vi "Pressure Tapped wing.vi"() -> ()   [LabVIEW 2022 SP3]
uses:
  Anemometry/Anemometry Sub Vis/Controls/User_Specific_mode.ctl
  Anemometry/Anemometry Sub Vis/Gen Trav/Trav_mode.ctl
  Anemometry/Anemometry Sub Vis/Controls/Tunnel_Coordinates.ctl
  Anemometry/Anemometry Sub Vis/Controls/Save_Data.ctl
  Anemometry/Anemometry Sub Vis/Gen Trav/Spacing.ctl
  Anemometry/Anemometry Sub Vis/Controls/Multi_run_mode.ctl
  Anemometry/Anemometry Sub Vis/Gen Trav/Traverse_cluster.ctl
  ADAM Client/Sub VIs/ADAM Controls/Tunnel_speed_mode.ctl
panel:
  in  "Tunnel Speed":dbl
  in  "End Position (mm)":sgl
  in  "Angle of Attack":sgl format="%#.1f"
  in  "Zero Pressure Transducers":bool
  in  "Take Traverse Profile":bool
  out "Velocity Profile":cluster{dbl[], dbl[]}(graph)
  in  "stop":bool
  out "Currently on Point":i32
  in  "Measure Pressures\n(without Saving)":bool
  in  "Number of Points":i32
  in  "Start Position (mm)":sgl
  out "Z":dbl format="%#.0f"
  out "U Trav":dbl format="%.2f"
  out "Uref":dbl format="%.2f"
  out "Pressure Distribution over wing":cluster{dbl[], dbl[]}[](graph)
  in  "Averaging time (Sec)":dbl=5.0
  in  "Filename":path=path "\\\\surrey.ac.uk\\personal/HS103/m13602/Documents/Wing_Results/test1.xls"
  in  "Take Pressure Measurement":bool
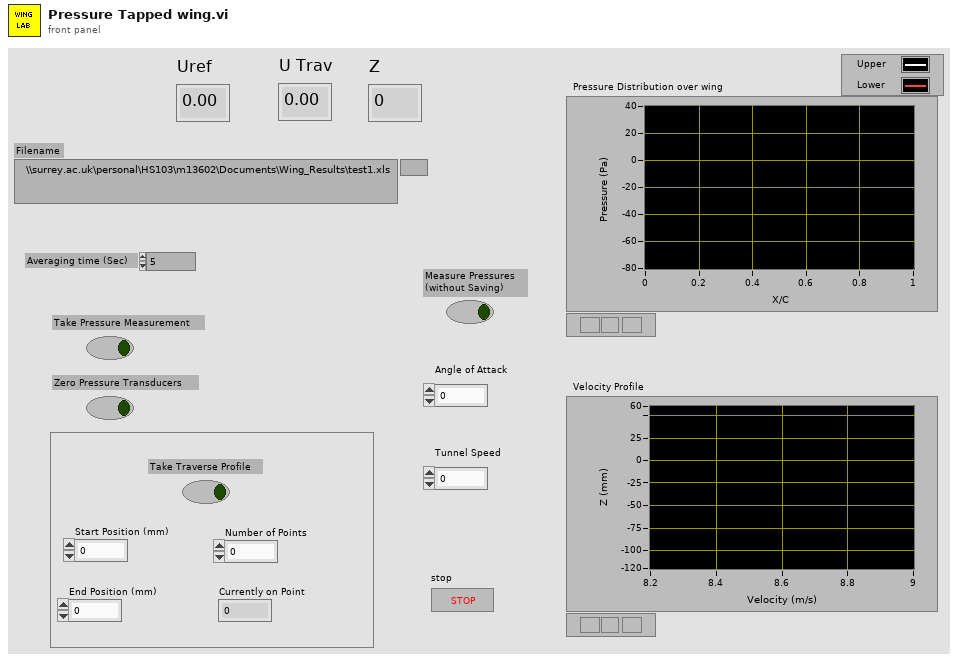
[diagram p1: front panel]
types:
  T1 = typedef "Tunnel_speed_mode.ctl" = enum16{"Set Speed", "Set Speed then wait", "Is tunnel speed allowable?"}
  T2 = typedef "Trav_mode.ctl" = enum16{"Move traverse", "Read traverse position", "Teach Position"}
  T3 = typedef "Tunnel_Coordinates.ctl" = enum16{"Work in Tunnel Coordinates", "Work in Model Coordinates"}
  T4 = typedef "User_Specific_mode.ctl" = enum16{"Check VI only", "Run VI"}
  T5 = typedef "Save_Data.ctl" = enum16{"Save No Data", "Save Data"}
  T6 = typedef "Traverse_cluster.ctl" = cluster{"Start X":sgl, "Start Y":sgl, "Start Z":sgl, "End X":sgl, "End Y":sgl, "End Z":sgl, "nPoints":i32, "Spacing":T7, "Filename":path, "Tunnel Speed":dbl, "Averaging time (mins)":dbl, "Extra Commands":string, "Carrier_1 Q (l/min)":dbl, "Carrier_2 Q (l/min)":dbl, "Trace Gas Concentration (%)":dbl, "Specific Arguments":string, "Comments":string, "Row No":i32, "Row Type Selector":T8, "EstCompl":string, "Row Duration (mins)":dbl, "nValidPoints":i32, "Meas Setup File":string}
  T7 = typedef "Spacing.ctl" = enum16{"Linear", "Log", "Gauss", "Specified", "N/A"}
  T8 = typedef "Multi_run_mode.ctl" = enum16{"Move Traverse Only", "Set Tunnel Speed Only", "Set Source Only", "Set Measurement Conditions", "Single Measurement", "Vertical Profile", "Lateral Profile", "Longitudinal Profile", "Multi-Axis Profile", "Explore Volume", "Auto Calibrate", "Meas Fast FID Bkgnd", "Check Beam Power", "Scanning Valve Measurement", "Run VI Named:", "Set ADAM Ch", "Wait (minutes)", "Send Message", "Synchronize With:", "Fall Back to this Row", "Turn Off Row Repeating", "Traverse 3D Volume", "Blank Row", "Jump to Fall Back Row"}
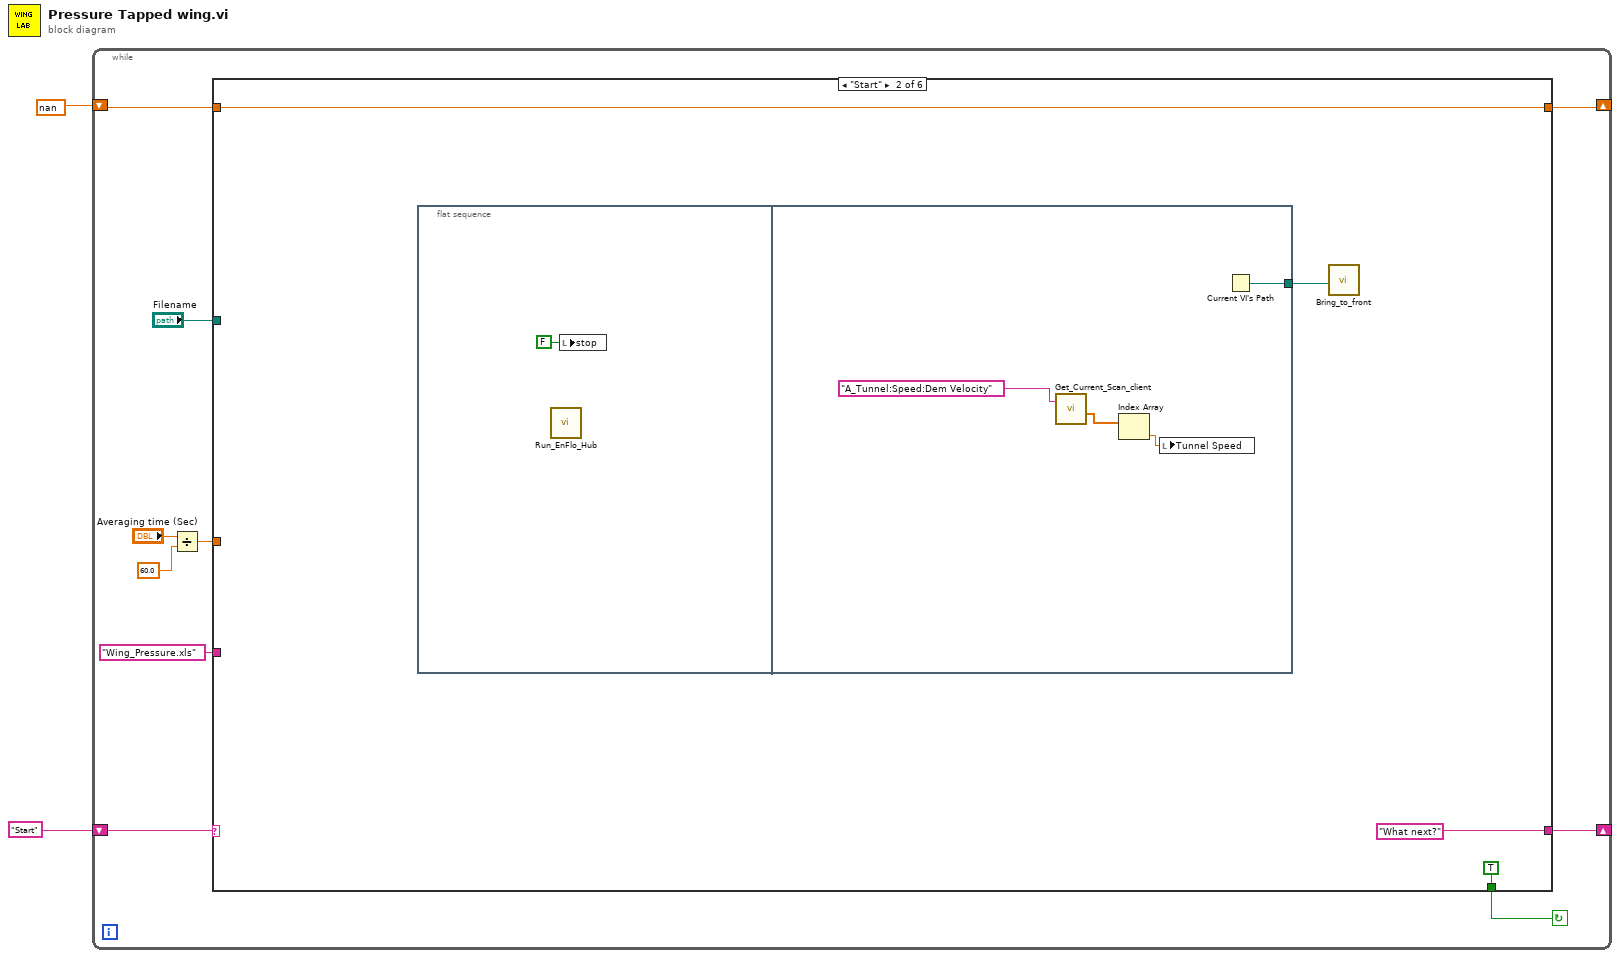
[diagram p0: block diagram]
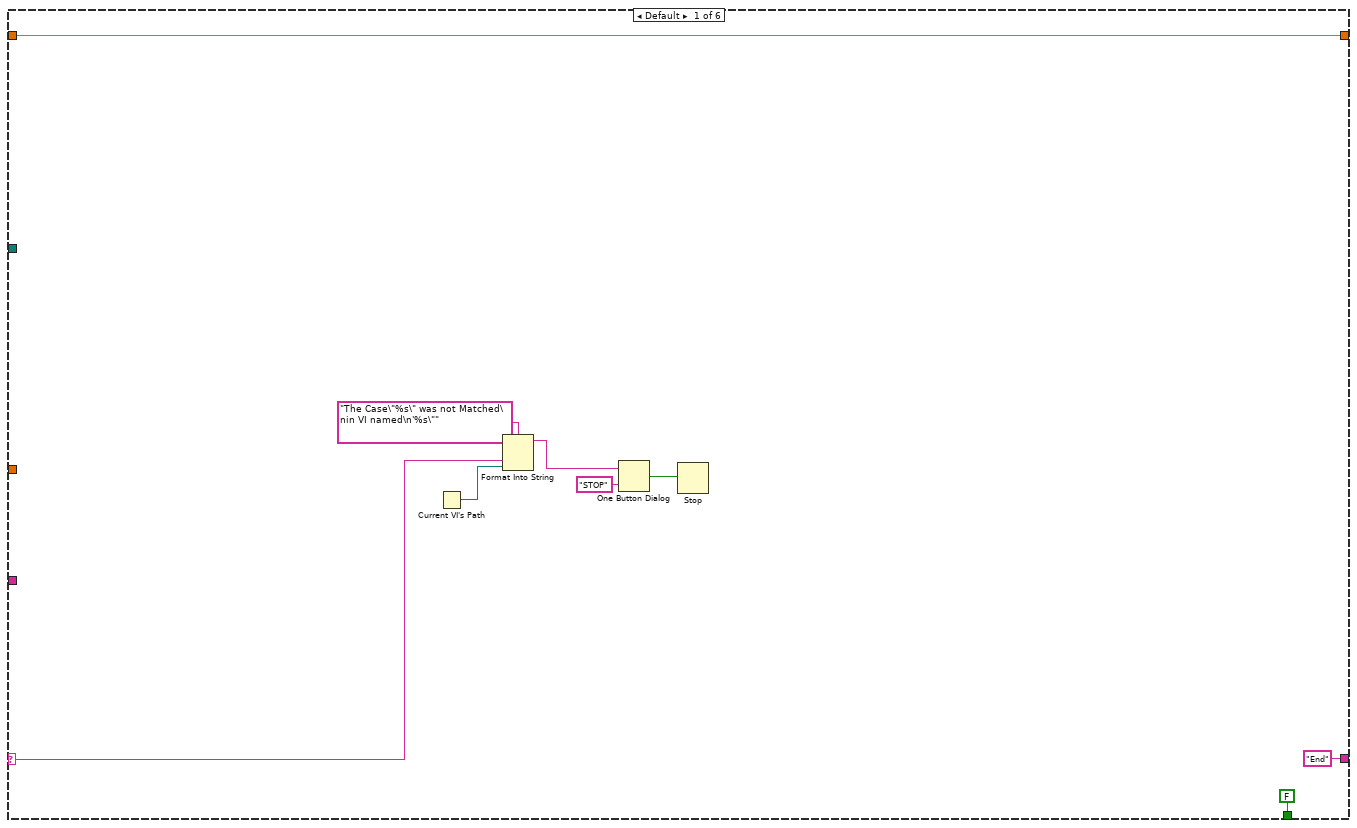
[diagram p2: hidden frame]
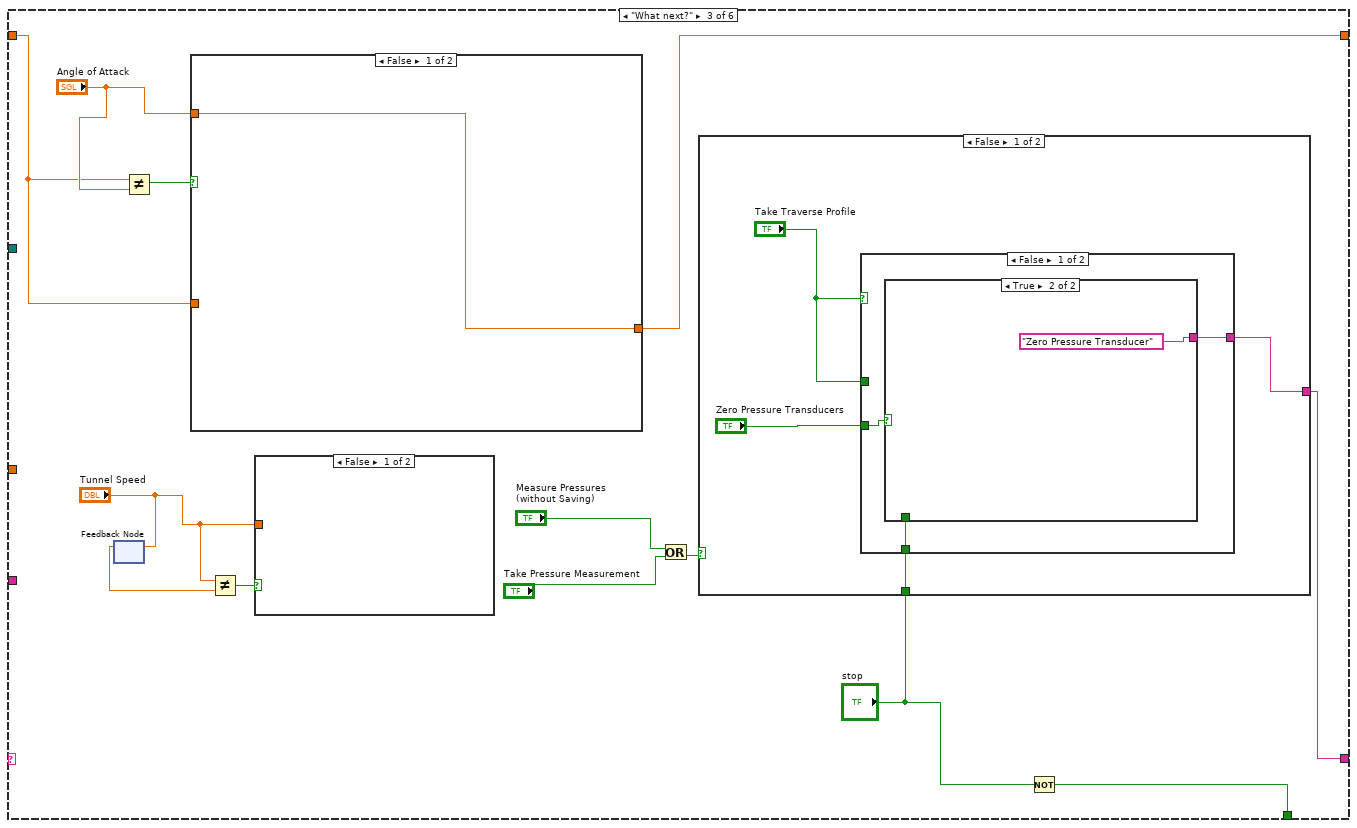
[diagram p3: hidden frame]
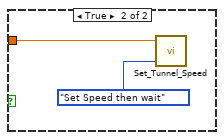
[diagram p4: hidden frame]
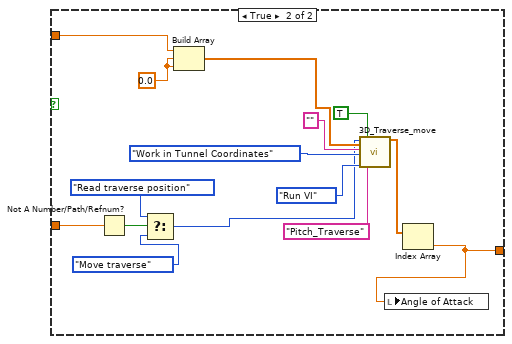
[diagram p5: hidden frame]
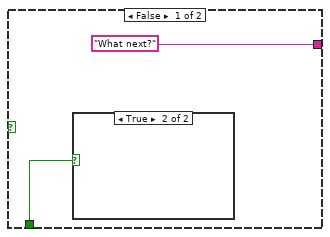
[diagram p6: hidden frame]
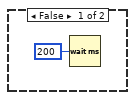
[diagram p7: hidden frame]
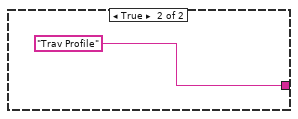
[diagram p8: hidden frame]
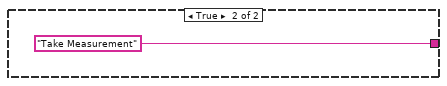
[diagram p9: hidden frame]
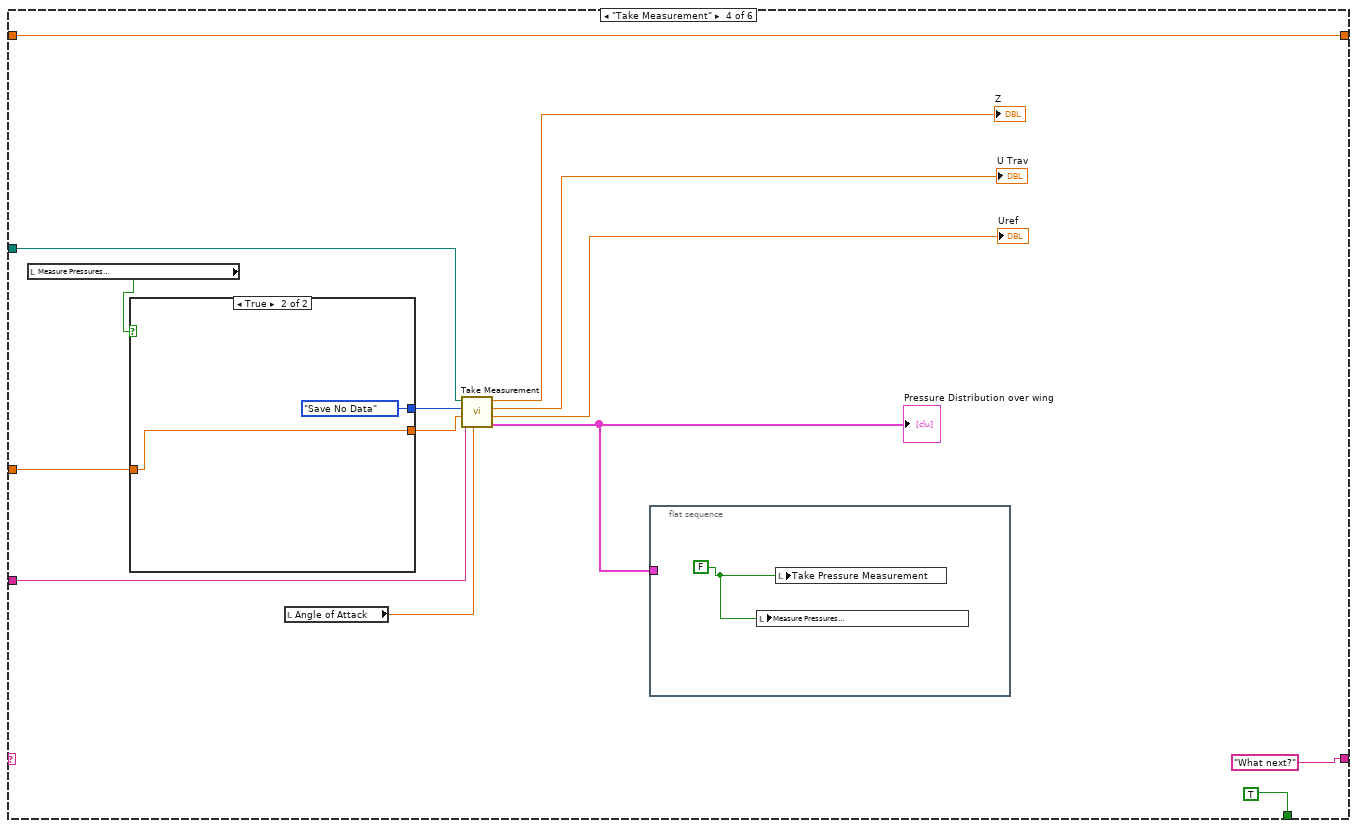
[diagram p10: hidden frame]
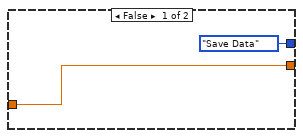
[diagram p11: hidden frame]
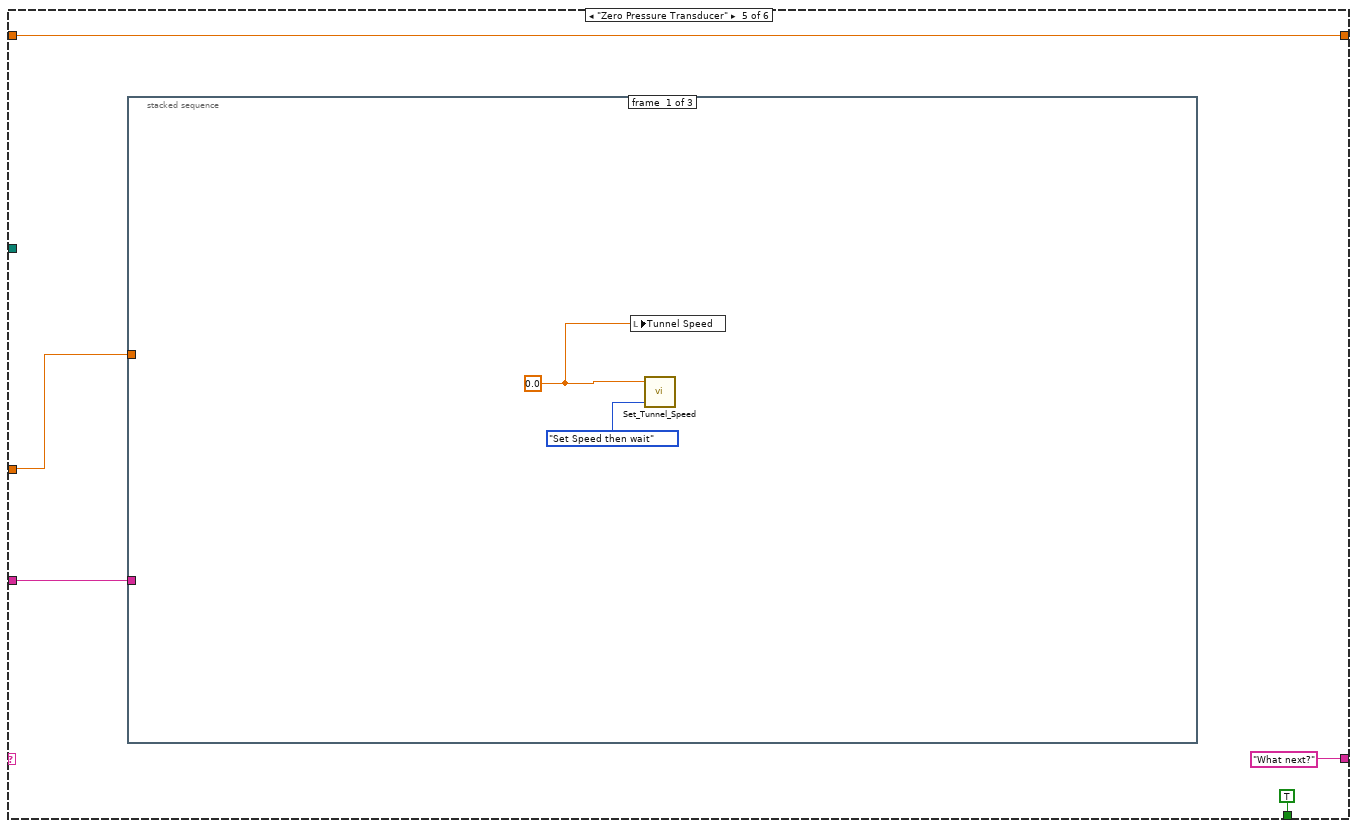
[diagram p12: hidden frame]
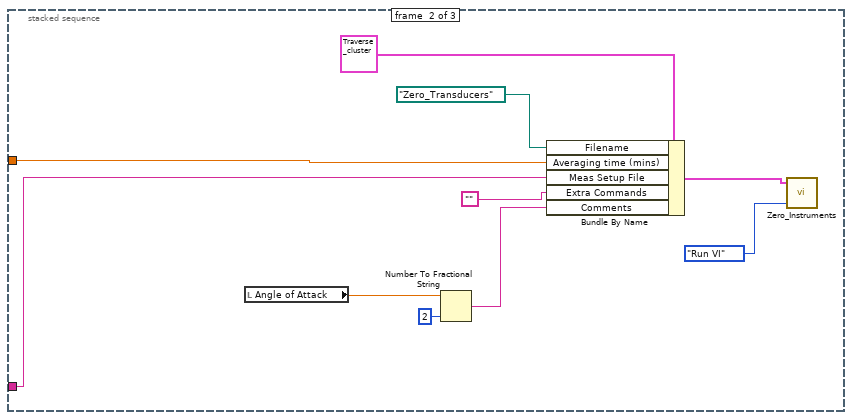
[diagram p13: hidden frame]
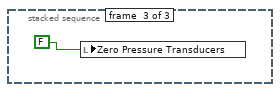
[diagram p14: hidden frame]
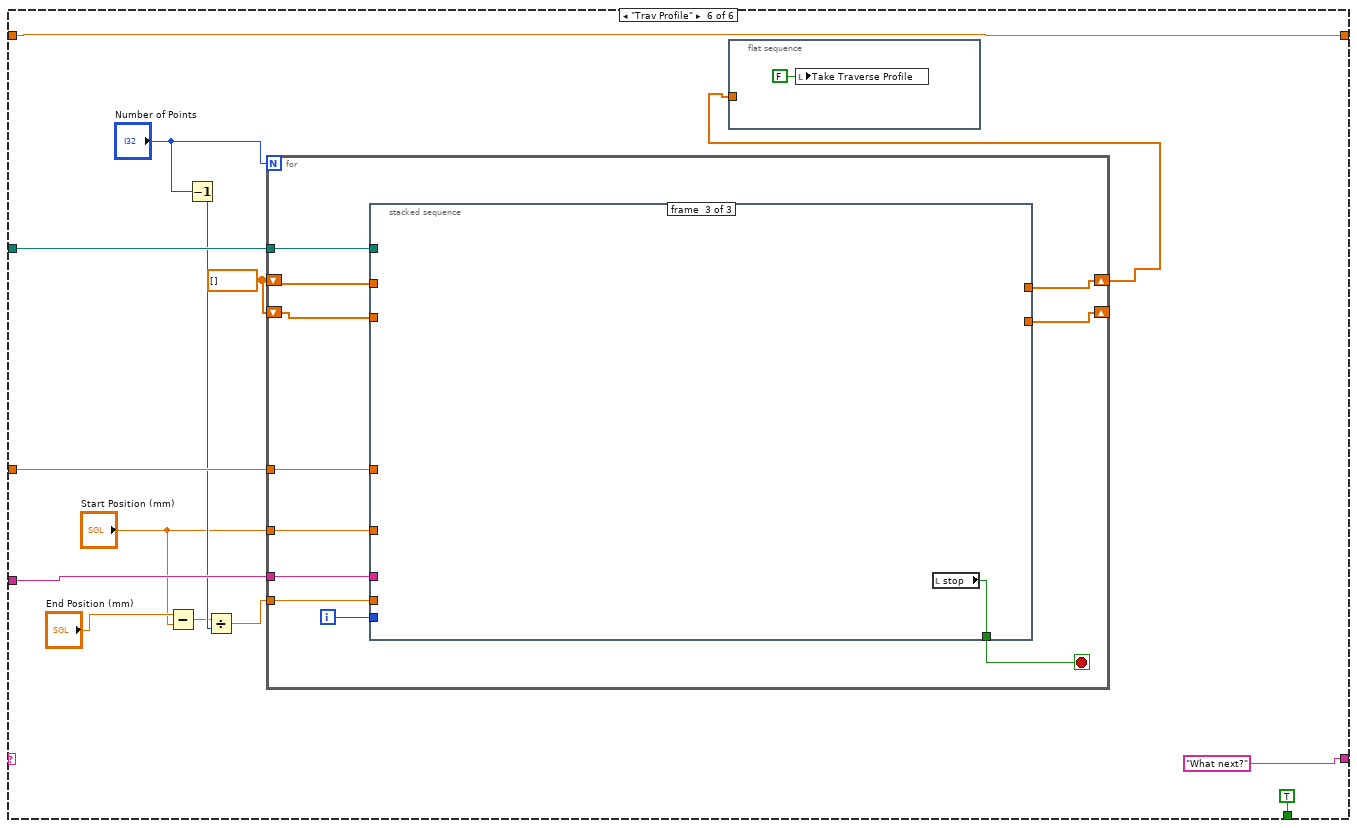
[diagram p15: hidden frame]
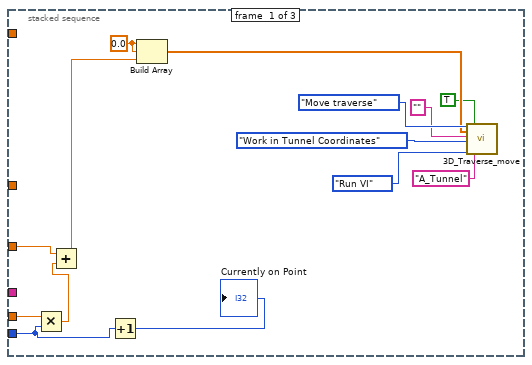
[diagram p16: hidden frame]
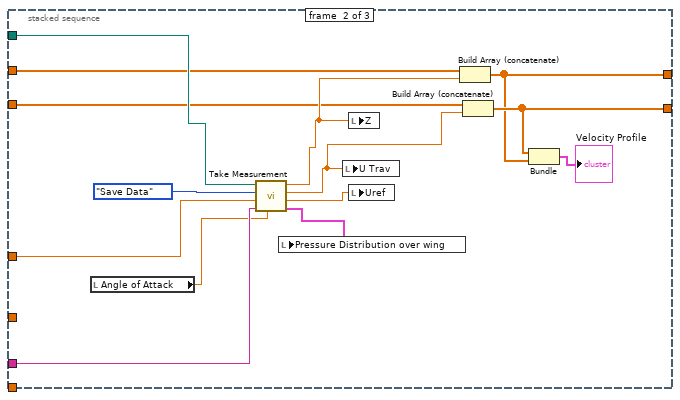
[diagram p17: hidden frame]
diagram:
  n1 = while {
    shift-right: [w6] -> _
    shift-left: "Start" -> [w11]
    shift-right: [w4] -> _
    shift-left: sgl nan -> [w3]
    stop <- w12 continue-if-true
    n2 = Divide(x="Averaging time (Sec)", y=60.0) -> (x/y=w7:dbl)
    n3 = case shown="\"Start\"" w11 {
      selector: w11 -> [w16 _ _ _ _ _]
      tunnel: [FALSE ("Stop Button") TRUE ("Stop Button") w43 TRUE ("Stop Button") TRUE ("Stop Button") TRUE ("Stop Button")] -> w12
      tunnel: "Filename" -> [_ _ _ w84 _ w125]
      tunnel: w7 -> [_ _ _ w79 w94 w124]
      tunnel: ["End" "What next?" w39 "What next?" "What next?" "What next?"] -> w6
      tunnel: "Wing_Pressure.xls" ("Setup filename") -> [_ _ _ w78 w98 w120]
      tunnel: [w13 w22 w31 w76 w95 w112] -> w4
      tunnel: w3 -> [w13 w22 w35 w76 w95 w112]
      frame Default {
        n4 = Current VI's Path() -> (path=w21:path)
        n5 = Format Into String(format string="The Case\"%s\" was not Matched\nin VI named\n'%s\"" ("Format String"), w16, w21) -> (resulting string=w18:string)  [unwired: 2 in, 1 out]
        n6 = One Button Dialog(message=w18, button name ("OK")="STOP") -> (true=w20:bool)
        n7 = Stop(stop? (T)=w20) -> ()
      }
      frame "Start" {
        n8 = flat-sequence {
          tunnel: [w30] -> w23
          frame #0 {
            n9 = call "Run_EnFlo_Hub.vi"() -> ()  [unwired: 7 in, 1 out]
            n10 = local write "stop"(FALSE ("stop")) -> ()
          }
          frame #1 {
            n11 = call "Get_Current_Scan_client.vi"("singleChannel"="A_Tunnel:Speed:Dem Velocity") -> ("Numerical Values"=w28:dbl[])  [unwired: 1 in, 3 out]
            n12 = Index Array(array=w28) -> (element=w27:dbl)  [unwired: 1 in]
            n13 = local write "Tunnel Speed"(w27) -> ()
            n14 = Current VI's Path() -> (path=w30:path)
          }
        }
        n15 = call "Bring_to_front.vi"("path"=w23) -> ()
      }
      frame "What next?" {
        n16 = feedback-in #1("Tunnel Speed") -> ()
        n17 = feedback #1() -> (w33:dbl)  [unwired: 1 in]
        n18 = Not Equal?(x=w35, y="Angle of Attack") -> (x != y?=w37:bool)
        n19 = case shown="False" w37 {
          tunnel: "Angle of Attack" -> [w46 w56]
          tunnel: w35 -> [_ w53]
          tunnel: [w46 w47] -> w31
          frame False {
          }
          frame True {
            w55 = sgl 0.0
            n20 = Not A Number/Path/Refnum?(number/path/refnum=w53) -> (NaN/Path/Refnum?=w48:bool)
            n21 = Select(t=Trav_mode."Read traverse position" ("Mode"), s=w48, f=Trav_mode."Move traverse" ("Mode")) -> (s? t:f=w50:T2)
            n22 = Build Array(w56, w55, w55) -> (w54:sgl[])
            n23 = call "3D_Traverse_move.vi"("Mode"=w50, "Position"=w54, "Extra command String"="", "Work in Tunnel Coordinates"=Tunnel_Coordinates."Work in Tunnel Coordinates", "Simulate/Run"=User_Specific_mode."Run VI", "Route Checking?"=TRUE, "Traverse name"="Pitch_Traverse") -> ("Trav Position achieved"=w49:sgl[])  [unwired: 9 in, 3 out]
            n24 = Index Array(array=w49) -> (element=w47:sgl)  [unwired: 1 in]
            n25 = local write "Angle of Attack"(w47) -> ()
          }
        }
        n26 = Not Equal?(x="Tunnel Speed", y=w33) -> (x != y?=w32:bool)
        n27 = case shown="False" w32 {
          tunnel: "Tunnel Speed" -> [_ w45]
          frame False {
          }
          frame True {
            n28 = call "Set_Tunnel_Speed.vi"("Mode"=Tunnel_speed_mode."Set Speed then wait", "Tunnel Velocity m/s"=w45) -> ()  [unwired: 2 in, 2 out]
          }
        }
        n29 = Or(x="Measure Pressures\n(without Saving)", y="Take Pressure Measurement") -> (x .or. y?=w40:bool)
        n30 = case shown="False" w40 {
          tunnel: [w64 "Take Measurement"] -> w39
          tunnel: "stop" -> [w63 _]
          frame False {
            n31 = case shown="False" "Take Traverse Profile" {
              tunnel: "Take Traverse Profile" -> [_ _]
              tunnel: [w68 "Trav Profile"] -> w64
              tunnel: w63 -> [w67 _]
              tunnel: "Zero Pressure Transducers" -> [w66 _]
              frame False {
                n32 = case shown="True" w66 {
                  tunnel: ["What next?" "Zero Pressure Transducer"] -> w68
                  tunnel: w67 -> [w69 _]
                  frame False {
                    n33 = case shown="True" w69 {
                      frame False {
                        n34 = Wait (ms)(milliseconds to wait=u32 200) -> ()  [unwired: 1 out]
                      }
                      frame True {
                      }
                    }
                  }
                  frame True {
                  }
                }
              }
              frame True {
              }
            }
          }
          frame True {
          }
        }
        n35 = Not(x="stop") -> (.not. x?=w43:bool)
      }
      frame "Take Measurement" {
        n36 = local read "Measure Pressures\n(without Saving)"() -> (w82:bool)
        n37 = case shown="True" w82 {
          tunnel: [Save_Data."Save Data" ("File") Save_Data."Save No Data" ("File")] -> w81
          tunnel: [w91 w92] -> w80
          tunnel: w79 -> [w91 w92]
          frame False {
          }
          frame True {
          }
        }
        n38 = local read "Angle of Attack"() -> (w75:sgl)
        n39 = call "Take Measurement.vi"("Angle of Attack"=w75, "Setup filename"=w78, "Averaging time (min)"=w80, "File"=w81, "Filename"=w84) -> ("Array"=w77:cluster{dbl[], dbl[]}[], "Uref"=→"Uref":dbl, "U Trav"=→"U Trav":dbl, "Z"=→"Z":dbl)  [unwired: 3 in]
        "Pressure Distribution over wing" <- w77
        n40 = flat-sequence {
          tunnel: w77 -> [_]
          frame #0 {
            w89 = FALSE ("Take Traverse Profile")
            n41 = local write "Measure Pressures\n(without Saving)"(w89) -> ()
            n42 = local write "Take Pressure Measurement"(w89) -> ()
          }
        }
      }
      frame "Zero Pressure Transducer" {
        n43 = stacked-sequence {
          tunnel: w98 -> [_ w105 _]
          tunnel: w94 -> [_ w101 _]
          frame #0 {
            w99 = 0.0 ("Tunnel Velocity m/s")
            n44 = local write "Tunnel Speed"(w99) -> ()
            n45 = call "Set_Tunnel_Speed.vi"("Mode"=Tunnel_speed_mode."Set Speed then wait", "Tunnel Velocity m/s"=w99) -> ()  [unwired: 2 in, 2 out]
          }
          frame #1 {
            n46 = local read "Angle of Attack"() -> (w102:sgl)
            n47 = Number To Fractional String(number=w102, precision (6)=i16 2) -> (F-format string=w107:string)  [unwired: 2 in]
            n48 = Bundle By Name(cluster=T6 {"Start X"=0.0, "Start Y"=0.0, "Start Z"=0.0, "End X"=0.0, "End Y"=0.0, "End Z"=0.0, "nPoints"=0, "Spacing"=enum."Linear", "Filename"=path "", "Tunnel Speed"=0.0, "Averaging time (mins)"=0.0, "Extra Commands"="", "Carrier_1 Q (l/min)"=0.0, "Carrier_2 Q (l/min)"=0.0, "Trace Gas Concentration (%)"=0.0, "Specific Arguments"="", "Comments"="", "Row No"=0, "Row Type Selector"=enum."Move Traverse Only", "EstCompl"="", "Row Duration (mins)"=0.0, "nValidPoints"=0, "Meas Setup File"=""} ("Traverse line In"), "Filename"=path "Zero_Transducers", "Averaging time (mins)"=w101, "Meas Setup File"=w105, "Extra Commands"="", "Comments"=w107) -> (w104:T6)
            n49 = call "Zero_Instruments.vi"("Mode"=User_Specific_mode."Run VI", "Traverse line In"=w104) -> ()  [unwired: 1 in, 3 out]
          }
          frame #2 {
            n50 = local write "Zero Pressure Transducers"(FALSE ("Take Traverse Profile")) -> ()
          }
        }
      }
      frame "Trav Profile" {
        w123 = dbl[] []
        n51 = Subtract(x="End Position (mm)", y="Start Position (mm)") -> (x-y=w116:sgl)
        n52 = Decrement(x="Number of Points") -> (x-1=w117:i32)
        n53 = Divide(x=w116, y=w117) -> (x/y=w113:sgl)
        n54 = for {
          N: "Number of Points" -> [_]
          tunnel: w125 -> [w137]
          tunnel: w124 -> [w136]
          tunnel: w113 -> [w134]
          tunnel: "Start Position (mm)" -> [w133]
          shift-right: [w131] -> w119
          shift-left: w123 -> [w132]
          shift-right: [w129] -> _
          shift-left: w123 -> [w130]
          tunnel: w120 -> [w128]
          i -> [w135]
          stop <- w127 stop-if-true
          n55 = stacked-sequence {
            tunnel: w137 -> [_ w163 _]
            tunnel: w136 -> [_ w161 _]
            tunnel: w135 -> [w140 _ _]
            tunnel: w134 -> [w146 _ _]
            tunnel: w133 -> [w144 _ _]
            tunnel: w132 -> [_ w160 _]
            tunnel: [_ w155 _] -> w131
            tunnel: w130 -> [_ w157 _]
            tunnel: [_ w156 _] -> w129
            tunnel: w128 -> [_ w153 _]
            tunnel: [_ _ w166] -> w127
            frame #0 {
              w142 = sgl 0.0 ("element")
              n56 = Multiply(x=w146, y=w140) -> (x*y=w145:sgl)
              n57 = Add(x=w144, y=w145) -> (x+y=w143:sgl)
              n58 = Increment(x=w140) -> (x+1=→"Currently on Point":i32)
              n59 = Build Array(w142, w142, w143) -> (w141:sgl[])
              n60 = call "3D_Traverse_move.vi"("Mode"=Trav_mode."Move traverse", "Position"=w141, "Extra command String"="", "Work in Tunnel Coordinates"=Tunnel_Coordinates."Work in Tunnel Coordinates", "Simulate/Run"=User_Specific_mode."Run VI", "Route Checking?"=TRUE, "Traverse name"="A_Tunnel") -> ()  [unwired: 9 in, 4 out]
            }
            frame #1 {
              n61 = local read "Angle of Attack"() -> (w152:sgl)
              n62 = call "Take Measurement.vi"("Angle of Attack"=w152, "Setup filename"=w153, "Averaging time (min)"=w161, "File"=Save_Data."Save Data", "Filename"=w163) -> ("Array"=w165:cluster{dbl[], dbl[]}[], "Uref"=w164:dbl, "U Trav"=w158:dbl, "Z"=w159:dbl)  [unwired: 3 in]
              n63 = local write "Pressure Distribution over wing"(w165) -> ()
              n64 = local write "U Trav"(w158) -> ()
              n65 = local write "Z"(w159) -> ()
              n66 = local write "Uref"(w164) -> ()
              n67 = Build Array (concatenate)(w160, w159) -> (w155:dbl[])
              n68 = Build Array (concatenate)(w157, w158) -> (w156:dbl[])
              n69 = Bundle(w156, w155) -> (→"Velocity Profile":cluster{dbl[], dbl[]})  [unwired: 1 in]
            }
            frame #2 {
              n70 = local read "stop"() -> (w166:bool)
            }
          }
        }
        n71 = flat-sequence {
          tunnel: w119 -> [_]
          frame #0 {
            n72 = local write "Take Traverse Profile"(FALSE ("Take Traverse Profile")) -> ()
          }
        }
      }
    }
  }
